vi "makeTcpFrame.vi"(8 "error in":errorcluster, 11 "String in":string) -> (0 "error out":errorcluster, 2 "size":i32, 3 "String out":string)   [LabVIEW 2018]
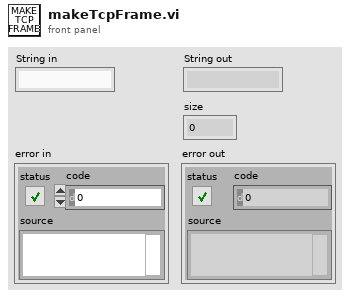
[diagram p1: front panel]
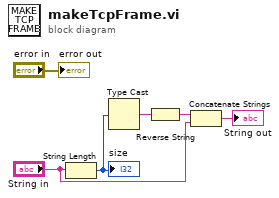
[diagram p0: block diagram]
diagram:
  n1 = String Length(string="String in") -> (length=w1:i32)
  "size" <- w1
  n2 = Type Cast(x=w1) -> (*(type *) &x=w3:string)  [unwired: 1 in]
  n3 = Reverse String(1:w3) -> (0:w2:string)
  n4 = Concatenate Strings(w2, "String in") -> (→"String out":string)
  "error out" <- "error in"
